vi "Reset.vi"(8 "Error In":errorcluster, 10 "CANopen Message":refnum<class "CANopen Response Message.lvclass">, 11 "reference in":refnum<class "Heartbeat.lvclass">) -> (0 "Error Out":errorcluster, 3 "reference out":refnum<class "Heartbeat.lvclass">)   [LabVIEW 2024, in "CANopen Master.lvlib" / "Heartbeat.lvclass"]
uses:
  Heartbeat.lvclass
  CANopen Response/CANopen Response Message.lvclass
  <vilib>/Utility/miscctls.llb/LVMapReplaceAction.ctl
  CANopen Message/CANopen Message.lvclass
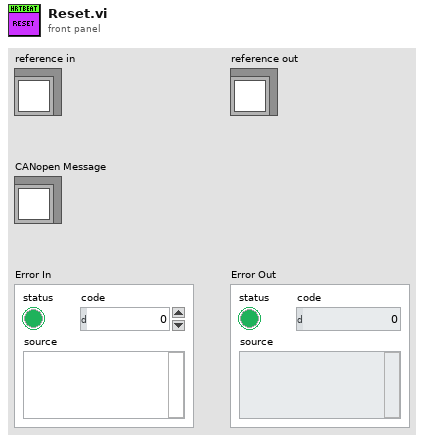
[diagram p1: front panel]
types:
  T1 = typedef "LVMapReplaceAction.ctl" = enum32{"Modify Entry only if found", "Add or Modify Entry", "Delete Entry"}
  T2 = typedef "CANopen Master.lvlib/Heartbeat.lvclass/ObjectAttributes.ctl" = cluster{"Heartbeats":map{u8, cluster{"Period":u16, "Timeout":u16, "Last Beat":refnum<class "Time Stamp.lvclass">}}}
  T3 = map{u8, cluster{"Period":u16, "Timeout":u16, "Last Beat":refnum<class "Time Stamp.lvclass">}}
  T4 = cluster{"Period":u16, "Timeout":u16, "Last Beat":refnum<class "Time Stamp.lvclass">}
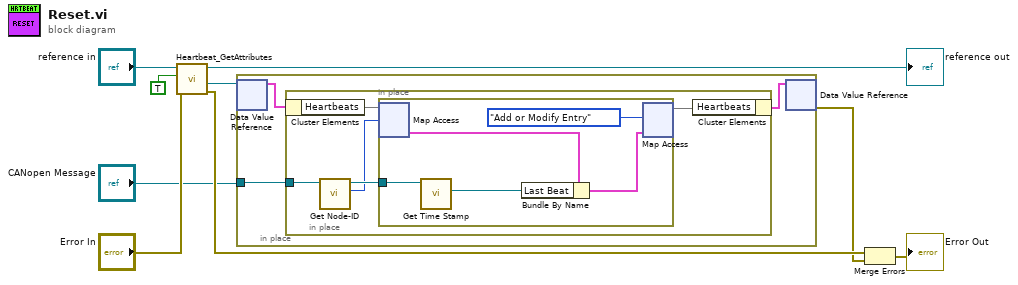
[diagram p0: block diagram]
diagram:
  n1 = call "Heartbeat_GetAttributes.vi"("Error In"="Error In", "OnlyGetDvrReference(False)"=TRUE, "reference in"="reference in") -> ("Error Out"=w8:errorcluster, "DataRef"=w3:refnum<data-value>, "reference out"=→"reference out":refnum<class "Heartbeat.lvclass">)  [unwired: 5 in, 1 out]
  n2 = in-place {
    in-place-border: "CANopen Message" -> [w10]
    n3 = in-place-dvr #1(w3) -> (w12:T2)  [unwired: 1 out]
    n4 = in-place {
      in-place-border: w10 -> [w15]
      n5 = in-place-cluster #2(w12) -> ("Heartbeats"=w17:T3)
      n6 = call "Get Node-ID.vi"("CANopen Message in"=w15) -> ("Node-ID"=w13:u8, "CANopen Message out"=w14:refnum<class "CANopen Response Message.lvclass">)  [unwired: 9 in]
      n7 = in-place {
        in-place-border: w14 -> [w19]
        n8 = in-place-map #3(w17, w13) -> (w22:T4)  [unwired: 1 in, 1 out]
        n9 = call "Get Time Stamp.vi"("CANopen Message in"=w19) -> ("Time Stamp"=w18:refnum<class "Time Stamp.lvclass">)  [unwired: 9 in, 1 out]
        n10 = Bundle By Name(cluster=w22, "Last Beat"=w18) -> (w21:T4)
        n11 = in-place-map #3(w21, LVMapReplaceAction."Add or Modify Entry" ("action")) -> (w16:T3)  [unwired: 2 out]
      }
      n12 = in-place-cluster #2("Heartbeats"=w16) -> (w11:T2)
    }
    n13 = in-place-dvr #1(w11) -> (w4:errorcluster)  [unwired: 1 out]
  }
  n14 = Merge Errors(w8, w4) -> (→"Error Out":errorcluster)
